vi "CreateTask.vi"(8 "error in":errorcluster, 11 "MainFGV_data":T1) -> (0 "error out":errorcluster, 3 "MainFGV_data out":T1)   [LabVIEW 2016]
uses:
  MainFGV_data.ctl
  CurrentMeter/CM_data.ctl
  CurrentMeter/CM_SerialNumber.ctl
  StrainGauge/SG_data.ctl
  <vilib>/DAQmx/create/channels.llb/DAQmx Create Channel (AI-Strain-Strain Gage).vi
  <vilib>/DAQmx/create/channels.llb/DAQmx Create Channel (AI-Current-Basic).vi
  <vilib>/DAQmx/configure/timing.llb/DAQmx Timing (Sample Clock).vi
  <resource>/objmgr/daqmx.rc
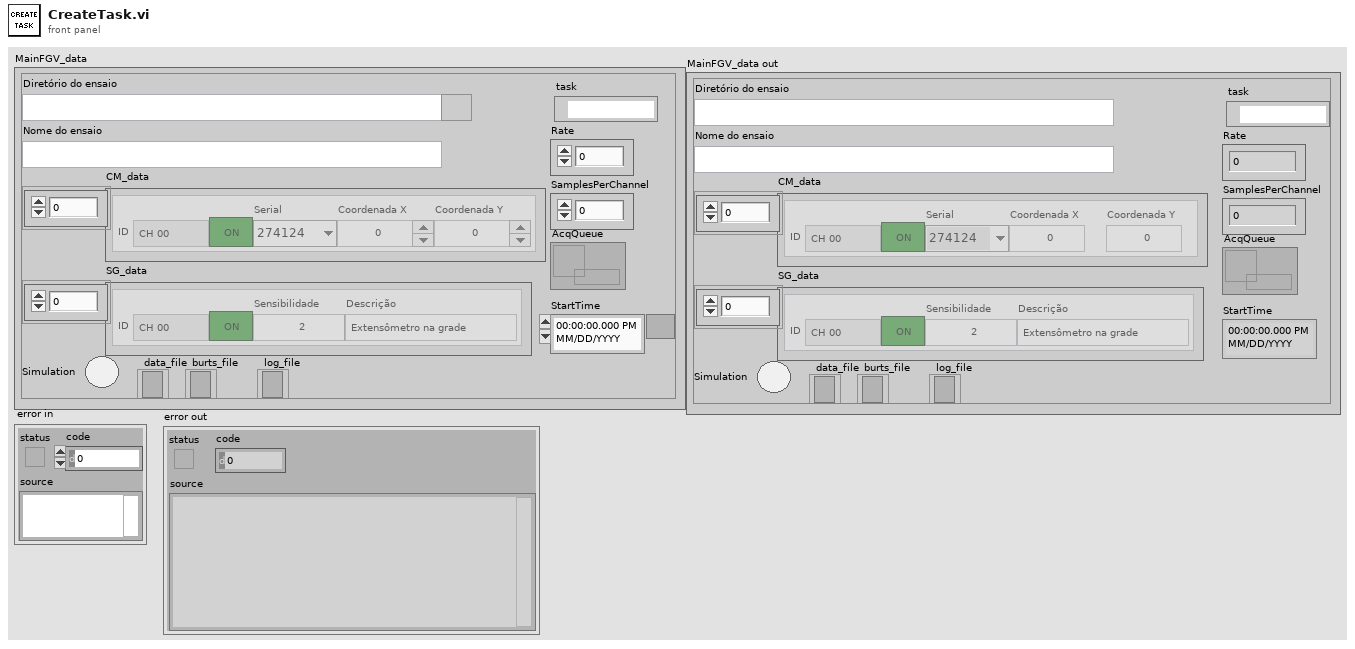
[diagram p1: front panel]
types:
  T1 = typedef "MainFGV_data.ctl" = cluster{"TestDir":path, "TestName":string, "CM_data":T2[], "SG_data":T4[], "Simulation":bool, "task":refnum<k21>, "data_file":refnum<file>, "burts_file":refnum<file>, "log_file":refnum<file>, "Rate":dbl, "SamplesPerChannel":dbl, "AcqQueue":refnum<queue>, "StartTime":timestamp}
  T2 = typedef "CM_data.ctl" = cluster{"Serial":T3, "Coordenada X":dbl, "Coordenada Y":dbl, "ID":string, "active":bool}
  T3 = typedef "CM_SerialNumber.ctl" = enum16{"274124", "274125", "274126", "274127", "274128"}
  T4 = typedef "SG_data.ctl" = cluster{"ID":string, "Sensibilidade":dbl, "Descrição":string, "active":bool}
  T5 = cluster{"gage factor":dbl, "nominal gage resistance":dbl, "poisson ratio":dbl}
  T6 = cluster{"strain configuration":i32, "lead wire resistance":dbl, "initial bridge voltage":dbl, "voltage excitation source":i32, "voltage excitation value":dbl}
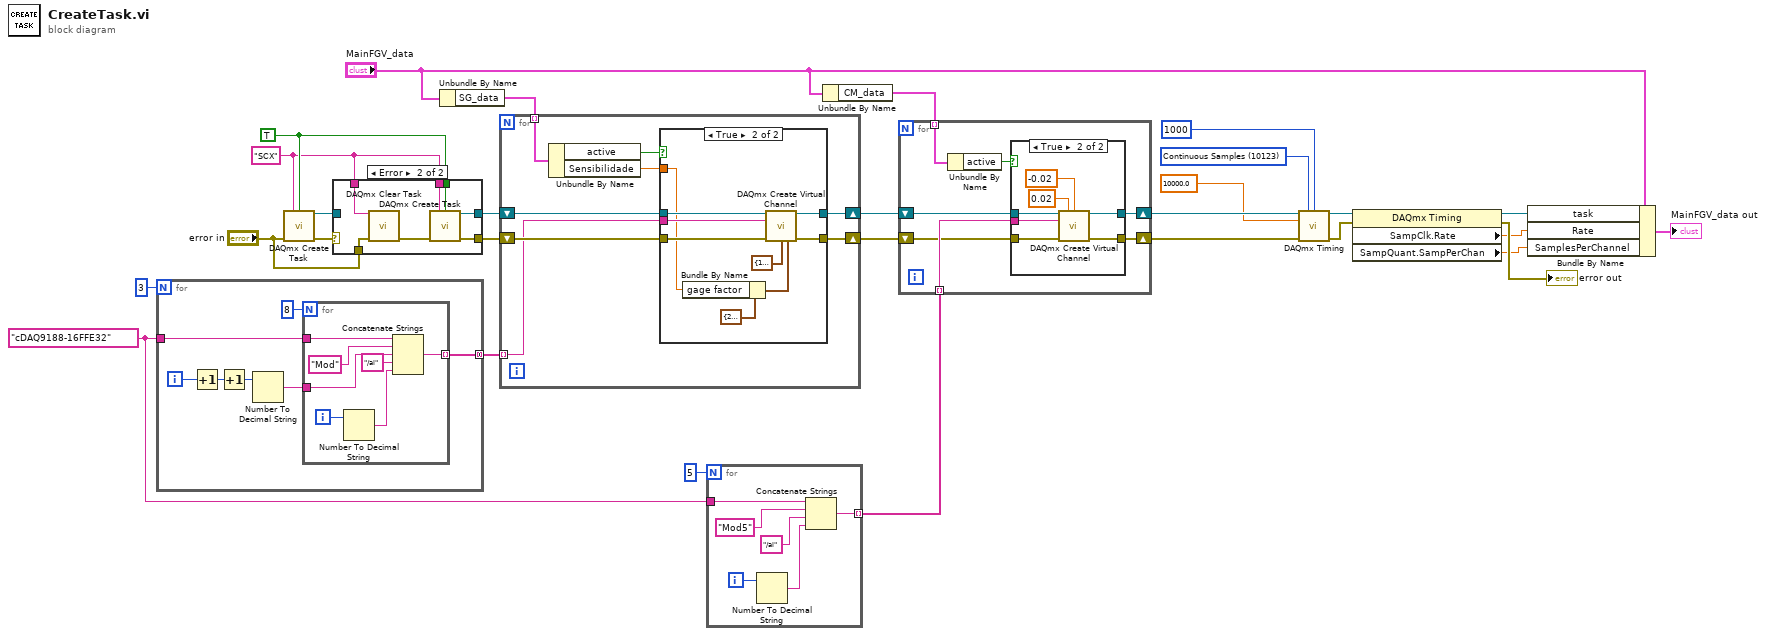
[diagram p0: block diagram]
diagram:
  w7 = 10123 items=["Finite Samples"=10178, "Continuous Samples"=10123, "Hardware Timed Single Point"=12522] ("sample mode")
  w9 = TRUE ("auto cleanup")
  w8 = "SCX" ("new task name")
  w17 = tag "cDAQ9188-16FFE32" ("DAQmx Device Name")
  n1 = for {
    N: 3 -> [_]
    tunnel: w17 -> [w36]
    tunnel: [w31] -> w28 mode=concatenating
    i -> [w34]
    n2 = Increment(x=w34) -> (x+1=w33:i32)
    n3 = Increment(x=w33) -> (x+1=w30:i32)
    n4 = Number To Decimal String(number=w30) -> (decimal integer string=w32:string)  [unwired: 1 in]
    n5 = for {
      N: 8 -> [_]
      tunnel: w36 -> [w43]
      tunnel: w32 -> [w41]
      tunnel: [w37] -> w31 mode=indexing
      i -> [w39]
      n6 = Number To Decimal String(number=w39) -> (decimal integer string=w38:string)  [unwired: 1 in]
      n7 = Concatenate Strings(w43, "Mod" ("string"), w41, "/ai" ("string"), w38) -> (w37:string)
    }
  }
  n8 = call <vilib>:"DAQmx Create Task.vi"("new task name"=w8, "auto cleanup"=w9, "error in"="error in") -> ("task out"=w13:refnum<k21>, "error out"=w14:errorcluster)  [unwired: 11 in]
  n9 = case shown="Error" w14 {
    selector: w14 -> [w44 _]
    tunnel: w13 -> [w45 _]
    tunnel: [w45 w47] -> w12
    tunnel: "error in" -> [_ w52]
    tunnel: [w44 w50] -> w10
    tunnel: w9 -> [_ w49]
    tunnel: w8 -> [_ w48]
    tunnel: w8 -> [_ w46]
    frame No Error {
    }
    frame Error {
      n10 = call <vilib>:"DAQmx Clear Task.vi"("task in"=w46, "error in"=w52) -> ("error out"=w51:errorcluster)  [unwired: 13 in]
      n11 = call <vilib>:"DAQmx Create Task.vi"("new task name"=w48, "auto cleanup"=w49, "error in"=w51) -> ("task out"=w47:refnum<k21>, "error out"=w50:errorcluster)  [unwired: 11 in]
    }
  }
  n12 = Unbundle By Name("MainFGV_data") -> ("SG_data"=w27:T4[])
  n13 = for {
    tunnel: w28 -> [w58] mode=indexing
    tunnel: w27 -> [w57] mode=indexing
    shift-right: [w54] -> w23
    shift-left: w12 -> [w60]
    shift-right: [w53] -> w22
    shift-left: w10 -> [w59]
    n14 = Unbundle By Name(w57) -> ("active"=w56:bool, "Sensibilidade"=w55:dbl)
    n15 = case shown="True" w56 {
      tunnel: w60 -> [w62 w71]
      tunnel: w59 -> [w61 w70]
      tunnel: w58 -> [_ w69]
      tunnel: w55 -> [_ w66]
      tunnel: [w62 w64] -> w54
      tunnel: [w61 w63] -> w53
      frame False {
      }
      frame True {
        n16 = Bundle By Name(cluster=T5 {"gage factor"=2.0, "nominal gage resistance"=350.0, "poisson ratio"=0.3} ("strain gage information"), "gage factor"=w66) -> (w65:T5)
        n17 = call-poly <vilib>:"DAQmx Create Virtual Channel.vi"("task in"=w71, "physical channels"=w69, "error in"=w70, "bridge information"=T6 {"strain configuration"=10271, "lead wire resistance"=0.0, "initial bridge voltage"=0.0, "voltage excitation source"=10200, "voltage excitation value"=3.3}, "strain gage information"=w65) -> ("task out"=w64:refnum<k21>, "error out"=w63:errorcluster)  [unwired: 9 in]
      }
    }
  }
  n18 = for {
    N: 5 -> [_]
    tunnel: [w73] -> w25 mode=indexing
    tunnel: w17 -> [w72]
    i -> [w75]
    n19 = Number To Decimal String(number=w75) -> (decimal integer string=w74:string)  [unwired: 1 in]
    n20 = Concatenate Strings(w72, "Mod5" ("string"), "/ai" ("string"), w74) -> (w73:string)
  }
  n21 = Unbundle By Name("MainFGV_data") -> ("CM_data"=w24:T2[])
  n22 = for {
    tunnel: w25 -> [w82] mode=indexing
    tunnel: w24 -> [w84] mode=indexing
    shift-right: [w78] -> w20
    shift-left: w23 -> [w81]
    shift-right: [w79] -> w21
    shift-left: w22 -> [w80]
    n23 = Unbundle By Name(w84) -> ("active"=w83:bool)
    n24 = case shown="True" w83 {
      tunnel: w82 -> [_ w93]
      tunnel: w81 -> [w86 w92]
      tunnel: w80 -> [w85 w91]
      tunnel: [w85 w90] -> w79
      tunnel: [w86 w89] -> w78
      frame False {
      }
      frame True {
        n25 = call-poly <vilib>:"DAQmx Create Virtual Channel.vi"("task in"=w92, "maximum value"=0.02, "minimum value"=-0.02, "physical channels"=w93, "error in"=w91) -> ("task out"=w89:refnum<k21>, "error out"=w90:errorcluster)  [unwired: 9 in]
      }
    }
  }
  n26 = call-poly <vilib>:"DAQmx Timing.vi"("task/channels in"=w20, "sample mode"=w7, "samples per channel"=1000, "rate"=10000.0, "error in"=w21) -> ("task out"=w6:refnum<k21>, "error out"=w5:errorcluster)  [unwired: 9 in]
  n27 = property class="DAQmx Timing"(reference=w6, error in=w5) -> (reference out=w3:refnum<k21>, error out=→"error out":errorcluster, "SampClk.Rate"=w2:dbl, "SampQuant.SampPerChan"=w1:dbl)
  n28 = Bundle By Name(cluster="MainFGV_data", "task"=w3, "Rate"=w2, "SamplesPerChannel"=w1) -> (→"MainFGV_data out":T1)
